vi "GUI Close Synchronization Objects.vi"(8 "error in (no error)":errorcluster, 11 "FOFB GUI":T1) -> (0 "error out":errorcluster)   [LabVIEW 2011, in "User Interface VIs.lvlib"]
uses:
  User Interface VIs.lvlib
  Types Definitions/Type FOFB GUI.ctl
  Types Definitions/Type FOFB Parameters.ctl
  Types Definitions/Type Network Configuration.ctl
  Types Definitions/Type FA Configuration.ctl
  Types Definitions/Type Response Matrix Measurement Configuration.ctl
  Types Definitions/Type Correction Algorithm Configuration.ctl
  Types Definitions/Type Acquisition Network Configuration.ctl
  Types Definitions/Type Actuation Network Configuration.ctl
  Types Definitions/Type Configuration Loop Mode.ctl
  Types Definitions/Type Configuration Data (GUI to Controller).ctl
  Types Definitions/Type Monitoring Data.ctl
  Types Definitions/Type Diagnostics Data.ctl
  Types Definitions/Type CPU Loads Array.ctl
  Types Definitions/Type CPU Loads.ctl
  Types Definitions/Type Diagnostics Sample.ctl
  Types Definitions/Type Monitoring Sample.ctl
  Type Definitions.lvlib
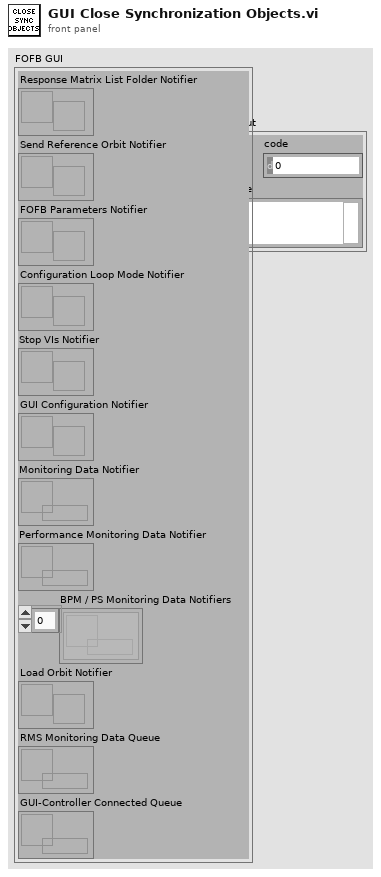
[diagram p1: front panel]
types:
  T1 = typedef "Type Definitions.lvlib/Type FOFB GUI.ctl" = cluster{"Response Matrix List Folder Notifier":refnum<notifier>, "Send Reference Orbit Notifier":refnum<notifier>, "FOFB Parameters Notifier":refnum<notifier>, "Configuration Loop Mode Notifier":refnum<notifier>, "Stop VIs Notifier":refnum<notifier>, "GUI Configuration Notifier":refnum<notifier>, "Monitoring Data Notifier":refnum<queue>, "Performance Monitoring Data Notifier":refnum<queue>, "BPM / PS Monitoring Data Notifiers":refnum<queue>[], "Load Orbit Notifier":refnum<notifier>, "RMS Monitoring Data Queue":refnum<queue>, "GUI-Controller Connected Queue":refnum<queue>}
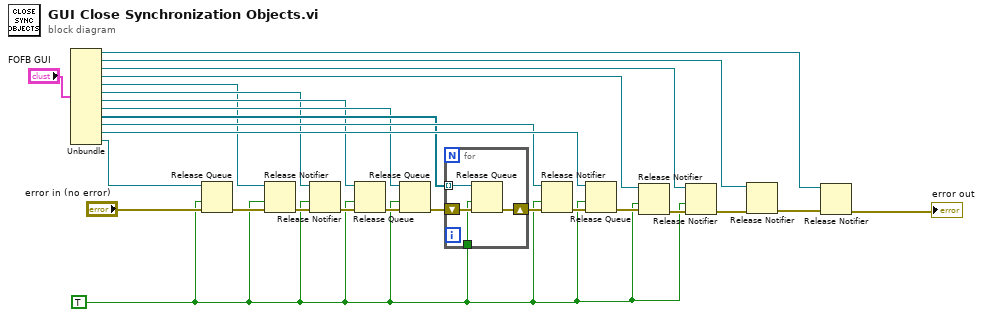
[diagram p0: block diagram]
diagram:
  w16 = TRUE ("force destroy? (F)")
  n1 = Unbundle("FOFB GUI") -> ("Response Matrix List Folder Notifier"=w1:refnum<notifier>, "Send Reference Orbit Notifier"=w4:refnum<notifier>, "FOFB Parameters Notifier"=w5:refnum<notifier>, "Configuration Loop Mode Notifier"=w6:refnum<notifier>, "Stop VIs Notifier"=w7:refnum<notifier>, "GUI Configuration Notifier"=w8:refnum<notifier>, "Monitoring Data Notifier"=w9:refnum<queue>, "Performance Monitoring Data Notifier"=w10:refnum<queue>, "BPM / PS Monitoring Data Notifiers"=w11:refnum<queue>[], "Load Orbit Notifier"=w12:refnum<notifier>, "RMS Monitoring Data Queue"=w13:refnum<queue>, "GUI-Controller Connected Queue"=w14:refnum<queue>)
  n2 = Release Queue(queue=w14, force destroy? (F)=w16, error in (no error)="error in (no error)") -> (error out=w19:errorcluster)  [unwired: 2 out]
  n3 = Release Notifier(notifier=w7, force destroy? (F)=w16, error in (no error)=w19) -> (error out=w26:errorcluster)  [unwired: 2 out]
  n4 = Release Notifier(notifier=w8, force destroy? (F)=w16, error in (no error)=w26) -> (error out=w25:errorcluster)  [unwired: 2 out]
  n5 = Release Queue(queue=w9, force destroy? (F)=w16, error in (no error)=w25) -> (error out=w24:errorcluster)  [unwired: 2 out]
  n6 = Release Queue(queue=w10, force destroy? (F)=w16, error in (no error)=w24) -> (error out=w23:errorcluster)  [unwired: 2 out]
  n7 = for {
    tunnel: w11 -> [w31] mode=indexing
    shift-right: [w29] -> w22
    shift-left: w23 -> [w30]
    tunnel: w16 -> [w28]
    n8 = Release Queue(queue=w31, force destroy? (F)=w28, error in (no error)=w30) -> (error out=w29:errorcluster)  [unwired: 2 out]
  }
  n9 = Release Notifier(notifier=w12, force destroy? (F)=w16, error in (no error)=w22) -> (error out=w21:errorcluster)  [unwired: 2 out]
  n10 = Release Queue(queue=w13, force destroy? (F)=w16, error in (no error)=w21) -> (error out=w17:errorcluster)  [unwired: 2 out]
  n11 = Release Notifier(notifier=w6, force destroy? (F)=w16, error in (no error)=w17) -> (error out=w18:errorcluster)  [unwired: 2 out]
  n12 = Release Notifier(notifier=w5, force destroy? (F)=w16, error in (no error)=w18) -> (error out=w15:errorcluster)  [unwired: 2 out]
  n13 = Release Notifier(notifier=w4, error in (no error)=w15) -> (error out=w3:errorcluster)  [unwired: 1 in, 2 out]
  n14 = Release Notifier(notifier=w1, error in (no error)=w3) -> (error out=→"error out":errorcluster)  [unwired: 1 in, 2 out]
